vi "步响应试验.vi"() -> ()   [LabVIEW 2013]
uses:
  <vilib>/Analysis/3filter.llb/Filter Passband Type.ctl
  <vilib>/Utility/config.llb/Read Key (String).vi
  <vilib>/Analysis/3filter.llb/Butterworth Filter (DBL).vi
  <vilib>/Analysis/NI_AALBase.lvlib
  <vilib>/Utility/config.llb/NI_LVConfig.lvlib
panel:
  out "波形图":dbl[][](graph) caption="当前试验模式：步响应试验"
  out "上升开始点":i32
  out "下降开始点":i32
  out "54%位置":dbl
  out "50%位置 2":dbl
  out "起点1":i32
  out "起点 2":i32
  out "起点 3":i32
  out "起点 4":i32
  out "过调时间正":dbl format="%.2f"
  out "全程时间正":dbl format="%.2f"
  out "最大过调量正":dbl
  out "过调时间回":dbl format="%.2f"
  out "全程时间回":dbl format="%.2f"
  out "最大过调量回":dbl
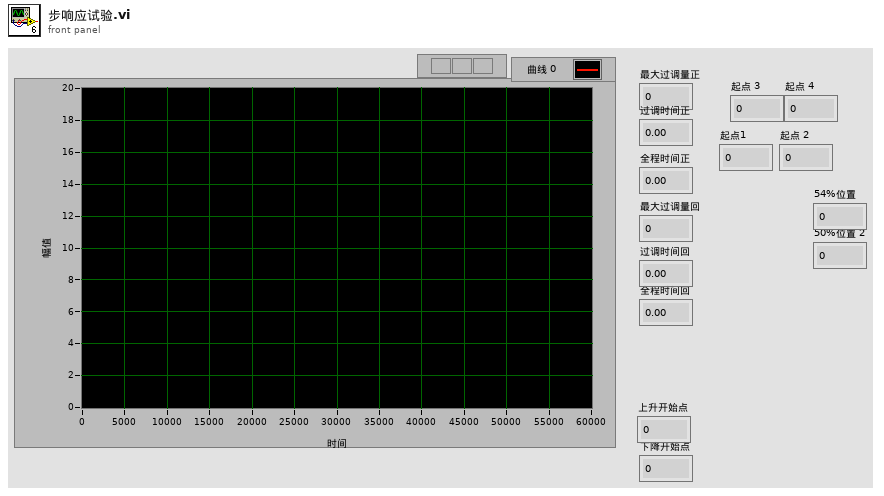
[diagram p1: front panel]
types:
  T1 = enum16{"open", "open or create", "create or replace", "create", "open (read-only)"}
  T2 = typedef "NI_AALBase.lvlib/Filter Passband Type.ctl" = enum32{"Lowpass", "Highpass", "Bandpass", "Bandstop"}
  T3 = typedef "NI_LVConfig.lvlib/Config Data RefNum.ctl" = refnum<k1>
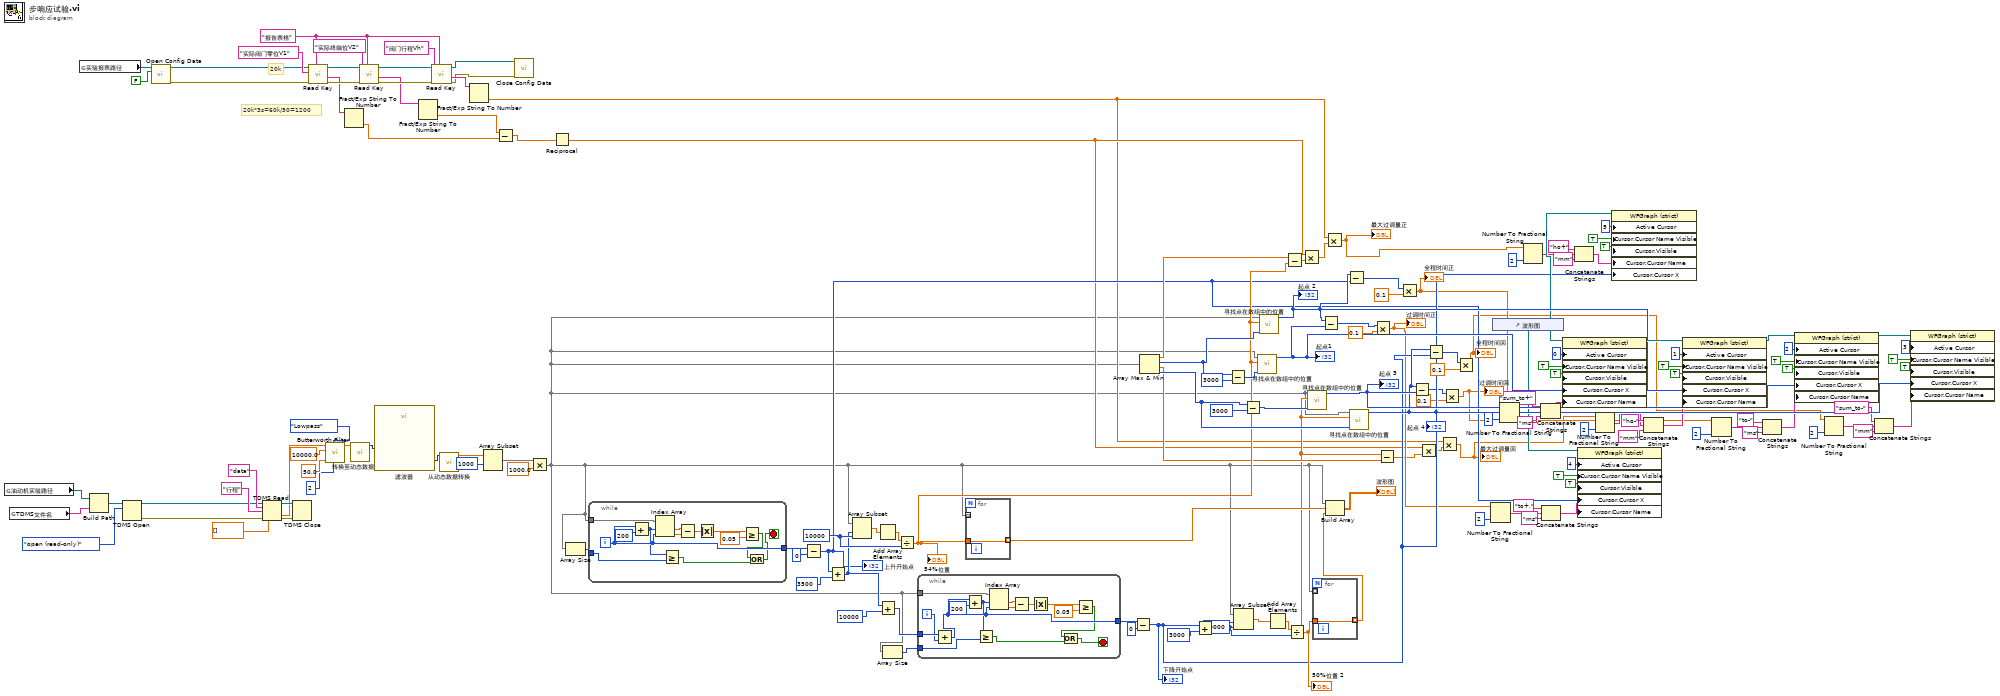
[diagram p0: block diagram]
diagram:
  w31 = "报告表格" ("section")
  w118 = 10000 ("长度")
  w130 = 10000 ("长度")
  # "20k*3s=60k/50=1200"
  # "20k"
  n1 = global read "油动机实验路径.vi" "油动机实验路径"() -> (w3:path)
  n2 = global read "TDMS文件名.vi" "TDMS文件名"() -> (w4:string)
  n3 = global read "实验报表路径.vi" "实验报表路径"() -> (w5:path)
  n4 = Build Path(base path=w3, name or relative path=w4) -> (appended path=w2:path)
  n5 = TDMS Open(10:T1."open (read-only)" ("operation (0:open)"), 11:w2) -> (0:w19:errorcluster, 3:w20:refnum<k34>)  [unwired: 5 in]
  n6 = call <vilib>:"Open Config Data.vi"("create file if necessary (T)"=FALSE, "configuration file path"=w5) -> ("error out"=w21:errorcluster, "refnum"=w22:T3)  [unwired: 7 in, 1 out]
  n7 = TDMS Read(0:w20, 5:"data" ("组名称输入"), 7:"行程" ("组名称输入"), 11:w19, 12:dbl[] []) -> (4:w148:refnum<k34>, 10:w142:dbl[], 15:w149:errorcluster)  [unwired: 3 in, 3 out]
  n8 = TDMS Close(8:w149, 11:w148) -> ()  [unwired: 2 out]
  n9 = call-poly <vilib>:"Read Key.vi"("section"=w31, "error in (no error)"=w21, "key"="实际阀门零位V1", "refnum"=w22) -> ("error out"=w35:errorcluster, "value"=w28:string, "refnum out"=w34:T3)  [unwired: 4 in, 1 out]
  n10 = call-poly <vilib>:"Butterworth Filter.vi"("order"=2, "filter type"=Filter_Passband_Type."Lowpass", "low cutoff freq: fl"=50.0, "sampling freq: fs"=10000.0, "X"=w142) -> ("Filtered X"=w143:dbl[])  [unwired: 3 in, 1 out]
  n11 = Fract/Exp String To Number(string=w28) -> (number=w24:dbl)  [unwired: 3 in, 1 out]
  n12 = call "转换至动态数据"("Array"=w143) -> ("Dynamic Data Type"=w140:dynamicdata)  [unwired: 3 in]
  n13 = call-poly <vilib>:"Read Key.vi"("section"=w31, "error in (no error)"=w35, "key"="实际终端位V2" ("default value"), "refnum"=w34) -> ("error out"=w33:errorcluster, "value"=w27:string, "refnum out"=w32:T3)  [unwired: 4 in, 1 out]
  n14 = call "滤波器"("Signal"=w140) -> ("Filtered Signal"=w139:dynamicdata)  [unwired: 9 in, 1 out]
  n15 = Fract/Exp String To Number(string=w27) -> (number=w25:dbl)  [unwired: 3 in, 1 out]
  n16 = call-poly <vilib>:"Read Key.vi"("section"=w31, "error in (no error)"=w33, "key"="阀门行程Vh", "refnum"=w32) -> ("error out"=w17:errorcluster, "value"=w26:string, "refnum out"=w18:T3)  [unwired: 4 in, 1 out]
  n17 = call "从动态数据转换"("Dynamic Data Type"=w139) -> ("Array"=w138:dbl[])  [unwired: 3 in]
  n18 = Fract/Exp String To Number(string=w26) -> (number=w9:dbl)  [unwired: 3 in, 1 out]
  n19 = Array Subset(array=w138, index=1000 ("索引")) -> (w136:dbl[])  [unwired: 1 in]
  n20 = Subtract(x=w25, y=w24) -> (x-y=w23:dbl)
  n21 = call <vilib>:"Close Config Data.vi"("error in (no error)"=w17, "refnum"=w18) -> ()  [unwired: 8 in, 2 out]
  n22 = Multiply(x=w136, y=1000.0) -> (x*y=w7:dbl[])
  n23 = Reciprocal(x=w23) -> (1/x=w10:dbl)
  n24 = Array Size(array=w7) -> (size(s)=w8:i32)
  n25 = while {
    tunnel: w7 -> [w166]
    tunnel: [w161] -> w134
    tunnel: w8 -> [w157]
    i -> [w161]
    stop <- w154 stop-if-true
    n26 = Add(x=w161, y=200) -> (x+y=w158:i32)
    n27 = Index Array(array=w166, index #1=w158, index #2=w161) -> (element #1=w165:dbl, element #2=w160:dbl)
    n28 = Greater Or Equal?(x=w158, y=w157) -> (x >= y?=w155:bool)
    n29 = Subtract(x=w165, y=w160) -> (x-y=w164:dbl)
    n30 = Absolute Value(x=w164) -> (abs(x)=w163:dbl)
    n31 = Greater Or Equal?(x=w163, y=0.05) -> (x >= y?=w156:bool)
    n32 = Or(x=w156, y=w155) -> (x .or. y?=w154:bool)
  }
  n33 = Subtract(x=w134, y=0) -> (x-y=w79:i32)
  "上升开始点" <- w79
  n34 = Add(x=w79, y=3500) -> (x+y=w127:i32)
  n35 = Array Subset(array=w7, index=w127, length=w130) -> (w132:dbl[])
  n36 = Add Array Elements(numeric array=w132) -> (sum=w131:dbl)
  n37 = Add(x=w127, y=10000 ("长度")) -> (x+y=w125:i32)
  n38 = Array Size(array=w7) -> (size(s)=w6:i32)
  n39 = Divide(x=w131, y=w130) -> (x/y=w109:dbl)
  "54%位置" <- w109
  n40 = while {
    tunnel: w7 -> [w181]
    tunnel: [w172] -> w124
    tunnel: w125 -> [w174]
    tunnel: w6 -> [w170]
    i -> [w173]
    stop <- w167 stop-if-true
    n41 = Add(x=w174, y=w173) -> (x+y=w172:i32)
    n42 = Add(x=w172, y=200) -> (x+y=w169:i32)
    n43 = Greater Or Equal?(x=w169, y=w170) -> (x >= y?=w171:bool)
    n44 = Index Array(array=w181, index #1=w169, index #2=w172) -> (element #1=w180:dbl, element #2=w176:dbl)
    n45 = Subtract(x=w180, y=w176) -> (x-y=w179:dbl)
    n46 = Absolute Value(x=w179) -> (abs(x)=w178:dbl)
    n47 = Greater Or Equal?(x=w178, y=0.05) -> (x >= y?=w168:bool)
    n48 = Or(x=w168, y=w171) -> (x .or. y?=w167:bool)
  }
  n49 = for {
    tunnel: w7 -> [_] mode=indexing
    tunnel: w109 -> [w182]
    tunnel: [w182] -> w129 mode=indexing
  }
  n50 = Subtract(x=w124, y=0) -> (x-y=w80:i32)
  "下降开始点" <- w80
  n51 = Array Max & Min(array=w7) -> (max value=w110:dbl, max index (indices)=w114:i32, min value=w108:dbl, min index (indices)=w111:i32)
  n52 = Add(x=w80, y=3000) -> (x+y=w121:i32)
  n53 = Subtract(x=w114, y=3000) -> (x-y=w116:i32)
  n54 = Array Subset(array=w7, index=w121, length=w118) -> (w119:dbl[])
  n55 = Subtract(x=w111, y=3000) -> (x-y=w112:i32)
  n56 = call "寻找点在数组中的位置.vi"("偏移量"=w116, "x"=w109, "数组"=w7) -> ("起点"=w91:i32)  [unwired: 8 in]
  "起点1" <- w91
  n57 = call "寻找点在数组中的位置.vi"("偏移量"=w114, "x"=w109, "数组"=w7) -> ("起点"=w90:i32)  [unwired: 8 in]
  "起点 2" <- w90
  n58 = Add Array Elements(numeric array=w119) -> (sum=w120:dbl)
  n59 = Subtract(x=w110, y=w109) -> (x-y=w15:dbl)
  n60 = Divide(x=w120, y=w118) -> (x/y=w107:dbl)
  "50%位置 2" <- w107
  n61 = Multiply(x=w10, y=w15) -> (x*y=w16:dbl)
  n62 = call "寻找点在数组中的位置.vi"("偏移量"=w112, "x"=w107, "数组"=w7) -> ("起点"=w89:i32)  [unwired: 8 in]
  "起点 3" <- w89
  n63 = for {
    tunnel: w107 -> [w183]
    tunnel: [w183] -> w117 mode=indexing
    tunnel: w7 -> [_] mode=indexing
  }
  n64 = Subtract(x=w90, y=w91) -> (x-y=w73:i32)
  n65 = Multiply(x=w9, y=w16) -> (x*y=w14:dbl)
  "最大过调量正" <- w14
  n66 = Build Array(w7, w129, w117) -> (→"波形图":dbl[][])
  n67 = Subtract(x=w90, y=w79) -> (x-y=w71:i32)
  n68 = call "寻找点在数组中的位置.vi"("偏移量"=w111, "x"=w107, "数组"=w7) -> ("起点"=w88:i32)  [unwired: 8 in]
  "起点 4" <- w88
  n69 = Multiply(x=w73, y=0.1) -> (x*y=w60:dbl)
  "过调时间正" <- w60
  n70 = Subtract(x=w107, y=w108) -> (x-y=w12:dbl)
  n71 = Multiply(x=w71, y=0.1) -> (x*y=w54:dbl)
  "全程时间正" <- w54
  n72 = Subtract(x=w88, y=w89) -> (x-y=w75:i32)
  n73 = Multiply(x=w10, y=w12) -> (x*y=w13:dbl)
  n74 = Subtract(x=w88, y=w80) -> (x-y=w78:i32)
  n75 = Multiply(x=w9, y=w13) -> (x*y=w11:dbl)
  "最大过调量回" <- w11
  n76 = Multiply(x=w75, y=0.1) -> (x*y=w38:dbl)
  "过调时间回" <- w38
  n77 = Multiply(x=w78, y=0.1) -> (x*y=w37:dbl)
  "全程时间回" <- w37
  n78 = Number To Fractional String(number=w60, precision (6)=i16 2 ("宽度(-)")) -> (F-format string=w63:string)  [unwired: 2 in]
  n79 = control-ref of="波形图"() -> (w81:refnum<vi>)
  n80 = Number To Fractional String(number=w54, precision (6)=i16 2 ("宽度(-)")) -> (F-format string=w58:string)  [unwired: 2 in]
  n81 = Number To Fractional String(number=w14, precision (6)=i16 2 ("宽度(-)")) -> (F-format string=w68:string)  [unwired: 2 in]
  n82 = Concatenate Strings("sum_to+" ("字符串"), w58, "ms" ("字符串")) -> (w55:string)
  n83 = Concatenate Strings("to+," ("光标.游标名"), w63, "ms" ("字符串")) -> (w61:string)
  n84 = property on="属性节点" class="WFGraph (strict)"(reference=w81, "Active Cursor"=u32 0 ("活动游标"), "Cursor.Cursor Name Visible"=TRUE ("光标.游标名可见"), "Cursor.Visible"=TRUE ("光标.可见"), "Cursor.Cursor X"=w91, "Cursor.Cursor Name"=w55) -> (reference out=w94:refnum<vi>)  [unwired: 1 in, 1 out]
  n85 = Concatenate Strings("ho+" ("光标.游标名"), w68, "mm" ("字符串")) -> (w66:string)
  n86 = property on="属性节点" class="WFGraph (strict)"(reference=w81, "Active Cursor"=u32 4 ("活动游标"), "Cursor.Cursor Name Visible"=TRUE ("光标.游标名可见"), "Cursor.Visible"=TRUE ("光标.可见"), "Cursor.Cursor X"=w79, "Cursor.Cursor Name"=w61) -> ()  [unwired: 1 in, 2 out]
  n87 = Number To Fractional String(number=w11, precision (6)=i16 2 ("宽度(-)")) -> (F-format string=w39:string)  [unwired: 2 in]
  n88 = property on="属性节点" class="WFGraph (strict)"(reference=w81, "Active Cursor"=u32 5 ("活动游标"), "Cursor.Cursor Name Visible"=TRUE ("光标.游标名可见"), "Cursor.Visible"=TRUE ("光标.可见"), "Cursor.Cursor Name"=w66, "Cursor.Cursor X"=w80) -> ()  [unwired: 1 in, 2 out]
  n89 = Concatenate Strings("ho-" ("字符串"), w39, "mm" ("字符串")) -> (w41:string)
  n90 = property on="属性节点" class="WFGraph (strict)"(reference=w94, "Active Cursor"=u32 1 ("活动游标"), "Cursor.Cursor Name Visible"=TRUE ("光标.游标名可见"), "Cursor.Visible"=TRUE ("光标.可见"), "Cursor.Cursor X"=w90, "Cursor.Cursor Name"=w41) -> (reference out=w93:refnum<vi>)  [unwired: 1 in, 1 out]
  n91 = Number To Fractional String(number=w38, precision (6)=i16 2 ("宽度(-)")) -> (F-format string=w49:string)  [unwired: 2 in]
  n92 = Concatenate Strings("to-" ("光标.游标名"), w49, "ms" ("字符串")) -> (w42:string)
  n93 = property on="属性节点" class="WFGraph (strict)"(reference=w93, "Active Cursor"=u32 2 ("活动游标"), "Cursor.Cursor Name Visible"=TRUE ("光标.游标名可见"), "Cursor.Visible"=TRUE ("光标.可见"), "Cursor.Cursor X"=w89, "Cursor.Cursor Name"=w42) -> (reference out=w92:refnum<vi>)  [unwired: 1 in, 1 out]
  n94 = Number To Fractional String(number=w37, precision (6)=i16 2 ("宽度(-)")) -> (F-format string=w45:string)  [unwired: 2 in]
  n95 = Concatenate Strings("sum_to-" ("光标.游标名"), w45, "mm" ("字符串")) -> (w43:string)
  n96 = property on="属性节点" class="WFGraph (strict)"(reference=w92, "Active Cursor"=u32 3 ("活动游标"), "Cursor.Cursor Name Visible"=TRUE ("光标.游标名可见"), "Cursor.Visible"=TRUE ("光标.可见"), "Cursor.Cursor X"=w88, "Cursor.Cursor Name"=w43) -> ()  [unwired: 1 in, 2 out]
